vi "TestHarnessDPL-DetBoardOnly.vi"() -> ()   [LabVIEW 2025]
uses:
  <vilib>/Analysis/NI_AALBase.lvlib
  <userlib>/_OpenG.lib/time/time.llb/openg_time.lvlib
  <instrlib>/Detector SCPI/Detector SCPI.lvlib
  <vilib>/Analysis/1siggen.llb/Ramp Pattern by Delta.vi
  <instrlib>/Keithley 24XX/Keithley 24XX.lvlib
  <vilib>/Analysis/1siggen.llb/Ramp Pattern by Samples.vi
  <instrlib>/Keithley 648X Series/Keithley 648X Series.lvlib
  <vilib>/Analysis/NI_AALPro.lvlib
  <vilib>/Analysis/6fits.llb/Curve Fitting Criteria.ctl
  <vilib>/Utility/file.llb/Write Delimited Spreadsheet (DBL).vi
  <vilib>/Utility/file.llb/Write Delimited Spreadsheet (string).vi
panel:
  out "Array":dbl[][](array[numeric])
  out "BoardTemperature":dbl
  out "PicoAmmeter Resource":refnum<visa-resource-name>="Picoammeter"
  out "Searching":dbl[][](array[numeric])
  out "error out":errorcluster
  out "OpVsCurrent":cluster{"Ramp Pattern":dbl[], dbl[]}[](array[cluster])
  in  "Exit":bool
  in  "Measurement Mode":T1(tab)
  in  "test Results save directory":path
  in  "DetectorData":T2(array[cluster]) {"DAC Offset" min=1 max=4095 step=1}
  in  "SPI Clock":i64=10000000 format="%^.0e"
  in  "Oversample":i32=1 min=1 max=4096
  in  "Power":bool=TRUE
  in  "Detector VISA":refnum<visa-resource-name>="Detector_EGSE"
  out "Detector Resource":refnum<visa-resource-name>="COM4"
  out "Voltage (V)":dbl[](array[numeric])=[3.264, 0.0, 12.488, 12.77]
  out "Current (mA)":dbl[](array[numeric])=[0.0, 0.0, 21.6, -3.65]
  in  "ThrowAway":i32=100 min=1 max=10000
  out "Detector EGSE ID String":string="Aberystwyth University,Enfys Detector,#01,v0.5.0\r\n"
  in  "Current source":refnum<visa-resource-name>
  in  "Channel":u16(ring) items=["SWIR:High", "SWIR:Med", "SWIR:Low", "MWIR:High", "MWIR:Med", "MWIR:Low", "TRP:HSink", "TRP:SWIR"]
  in  "ReadMode":enum16{"Science", "Debug"}(ring)
  in  "Tab Control":T3(tab)
  out "Counts":dbl(graph)=160.194
  out "size":i32
  out "Elapsed(uS)":i32
  out "Mean Value (counts)":dbl
  out "rms (counts) 2":dbl=-2.7284841053187847e-12 format="%^.4g"
  out "Peak-to-Peak (counts)":dbl=0.0026870000001508743 format="%^.4g"
  in  "ResetVDACstats":bool
  out "Searching...":bool
  in  "Find Offset":bool
  in  "Target Counts":i32 min=0 max=4095
  in  "Tolerance":dbl
  in  "DAC Value":i32=2076 min=0 max=4095 step=1
  in  "Detector":u16(ring) items=["SWIR", "MWIR"]
  in  "Gain":u16(ring) items=["High", "Med", "Low"]
  in  "Export to Excel":bool
  in  "ResetScienceGraph":bool
  out "All Counts":T4(graph)
  out "Save FileName":string
  out "Temperature":dbl(graph)=160.194
  out "Waveform Chart":cluster{"output":i32, "output":i32}(graph)
  in  "Pause":bool
  out "XY Graph":cluster{dbl[], "subarray":dbl[]}(graph)
  in  "Detector 3":u16(ring) items=["SWIR", "MWIR"]
  in  "Gain 3":u16(ring) items=["High", "Med", "Low"]
  in  "trig":dbl=8.0 min=0.0 max=50.0
  in  "DetectorDAC":i32=2076 min=0 max=4095 step=1
  out "Output vs current":cluster{"Ramp Pattern":dbl[], dbl[]}[](graph)
  in  "ISweep":bool
  in  "NPoints":i32=10 min=10 max=10000 step=1
  in  "MaxCurrent":dbl=1e-11 min=1e-11 max=1e-06
  in  "MinCurrent":dbl=1e-12 min=-10.0 max=10.0
  in  "Detector 4":u16(ring) items=["SWIR", "MWIR"]
  in  "DecadeSweep":bool
  in  "Gain 4":u16(ring) items=["High", "Med", "Low"]
  out "slope (counts/nA)":dbl
  out "intercept":dbl
  out "residue":dbl
  out "Max Deviation (counts)":dbl
  in  "NumberDecades":i32
  in  "DAC":i32 min=0 max=4095 step=1
  in  "Modulation Steps":i32=2 min=2 max=1000 step=1
  in  "Modulation Max":dbl min=0.0 max=10.0
  in  "Modulation Min":dbl min=-10.0 max=10.0
  in  "SweepLight":bool
  in  "Detector 7":u16(ring) items=["SWIR", "MWIR"]
  out "Output vs Light":cluster{dbl[], dbl[]}[](graph)
  in  "Gain 2":u16(ring) items=["High", "Med", "Low"]
  in  "Abort 2":bool
  out "Output vs Light 2":cluster{dbl[], dbl[]}[](graph)
  in  "StopGathering":bool=TRUE
  in  "Detector 2":u16(ring) items=["SWIR", "MWIR"]
  out "PhotoDiode":dbl
  in  "millisecond multiple":u32
  in  "Manual LightSweep":bool
  in  "Tab Control 2":enum32{"Individual", "Science Mode"}(tab)
  out "VDAC Sweep":cluster{dbl[], dbl[]}[](graph)
  out "All Counts 2":cluster{"X-Data":dbl[], "SciData":dbl[]}[](graph)
  in  "SweepVDAC":bool
  in  "ISource":dbl min=-1e-06 max=1e-06
  in  "VDAC Step":i32=1 min=1 max=100
  in  "VDAC Max":i32 min=0 max=4095
  in  "VDAC Min":i32 min=0 max=4000
  in  "Channel":u16(ring) items=["SWIR", "MWIR"]
  in  "Abort SweepVDAC":bool
  in  "Step":bool
  in  "Delay 1 (ms)":i32
  in  "Current 2":dbl
  in  "Current 1":dbl
  out "Step Response":cluster{dbl[], "subarray":dbl[]}(graph)
  in  "chan (0)":i32
  out "exit":bool=TRUE
  # "3.3V supply"
  # "Heater"
  # "+12V Supply"
  # "-12V Supply"
  # "Pause button will halt collection and display.\nThis allows graph to be printed etc."
  # "Burst mode is intended to examine behaviour of the ADC\n\nA burst of readings is recorded on the EGSE and then gathered here."
  # "Light source modulated by USB205L working as voltage source connected to MOD input of LD250C\nreference photodiode monitored by 6846 picoammeter"
  # "Light source modulated by USB205L working as voltage source connected to MOD input of LD250C\nreference photodiode monitored by 6846 picoammeter"
  # "Set current to Current#1. Waits for Delay 1 to stabilise, then switches to current 2 and reads 1000 readings as fast as possible"
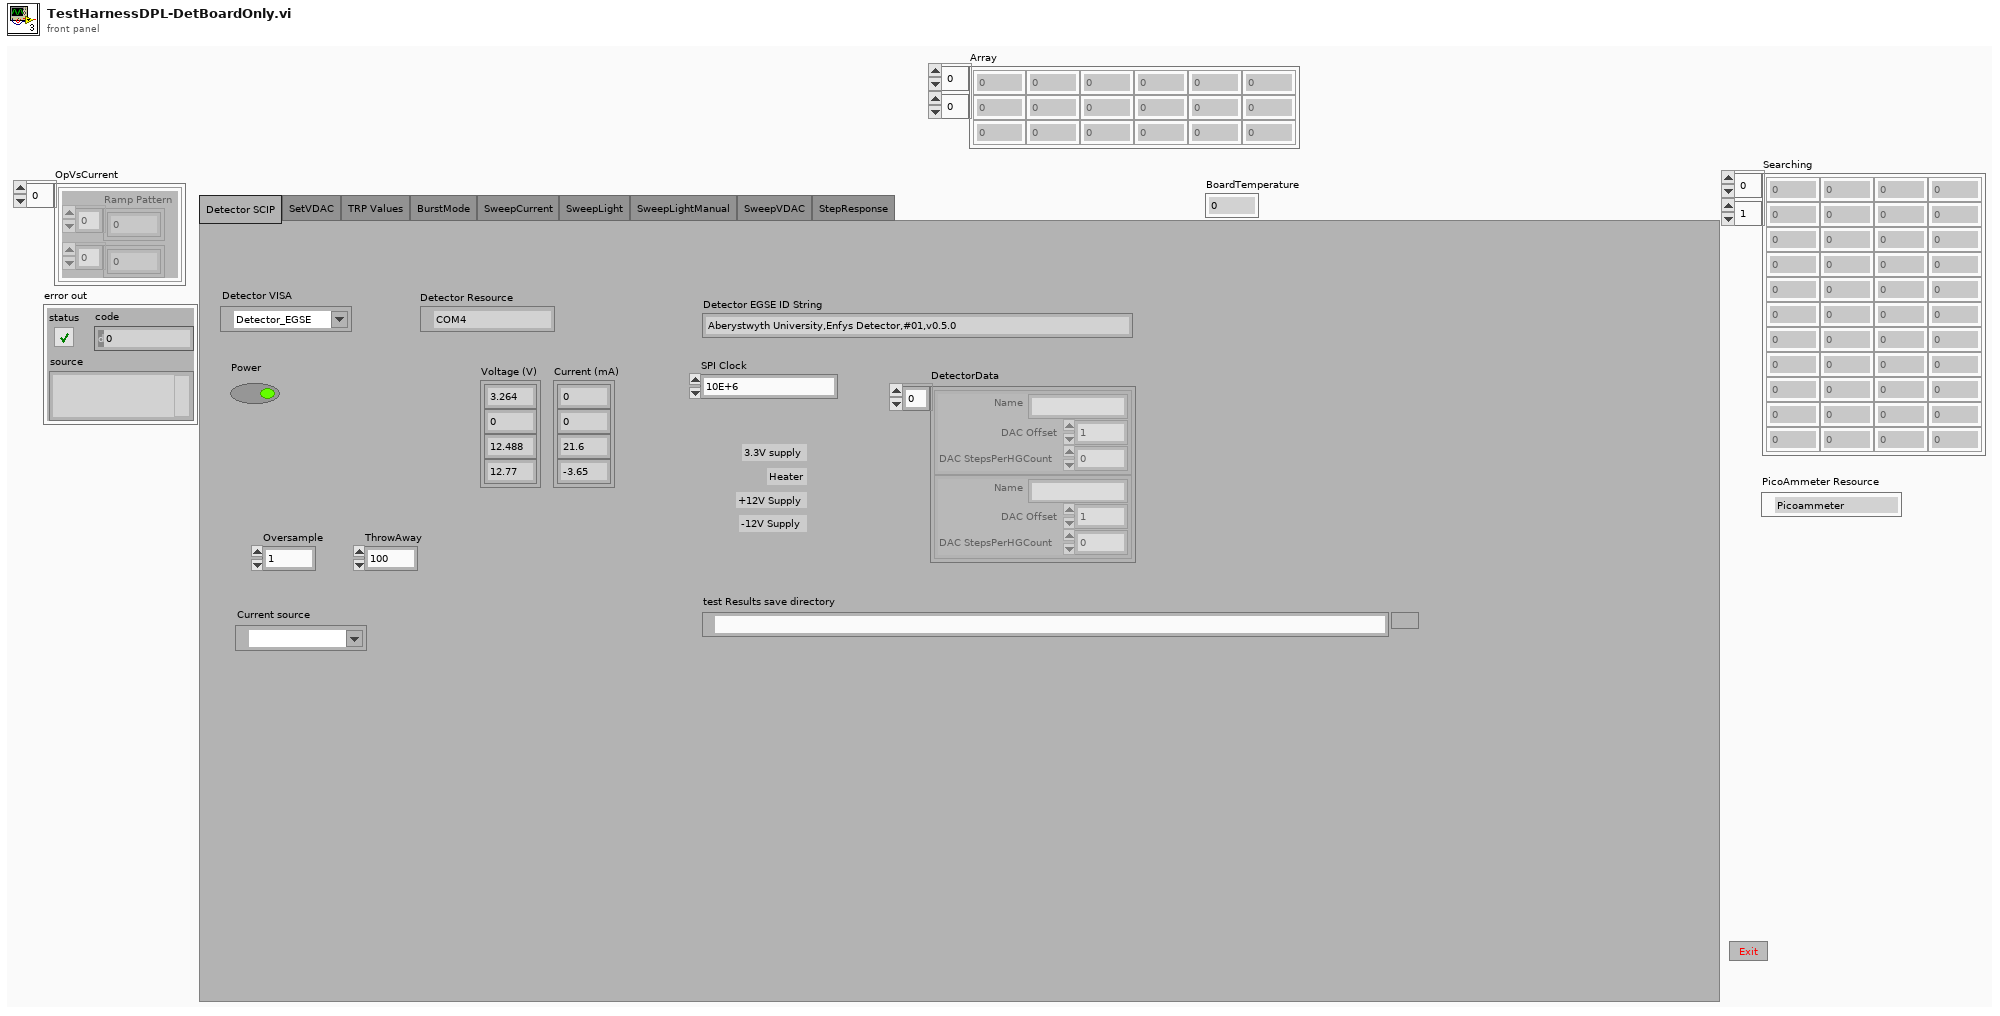
[diagram p1: front panel]
types:
  T1 = enum32{"Detector SCIP", "SetVDAC", "TRP Values", "BurstMode", "SweepCurrent", "SweepLight", "SweepLightManual", "SweepVDAC", "StepResponse"}
  T2 = cluster{"Name":string, "DAC Offset":i32, "DAC StepsPerHGCount":dbl}[]
  T3 = enum32{"Counts", "Science Packet", "Temperature"}
  T4 = cluster{"[0]":dbl, "[1]":dbl, "[2]":dbl, "[3]":dbl, "[4]":dbl, "[5]":dbl, "[6]":dbl, "[7]":dbl, "[8]":dbl, "[9]":dbl}
  T5 = cluster{"Baud Rate":u32, "Parity":u16, "Data Bits":u16, "Stop Bits":u16, "Flow Control":u16}
  T6 = cluster{"[0]":dbl, "[1]":dbl, "[2]":dbl, "[3]":dbl, "[4]":dbl, "[5]":dbl, "[6]":dbl, "[7]":dbl, "[8]":dbl, "[9]":dbl}[]
  T7 = cluster{"Name":string, "DAC Offset":i32, "DAC StepsPerHGCount":dbl}
  T8 = typedef "NI_AALPro.lvlib/Curve Fitting Criteria.ctl" = u16
  T9 = typedef "LVPointDoubleTypeDef.ctl" = cluster{"Cursor X":dbl, "Cursor Y":dbl}
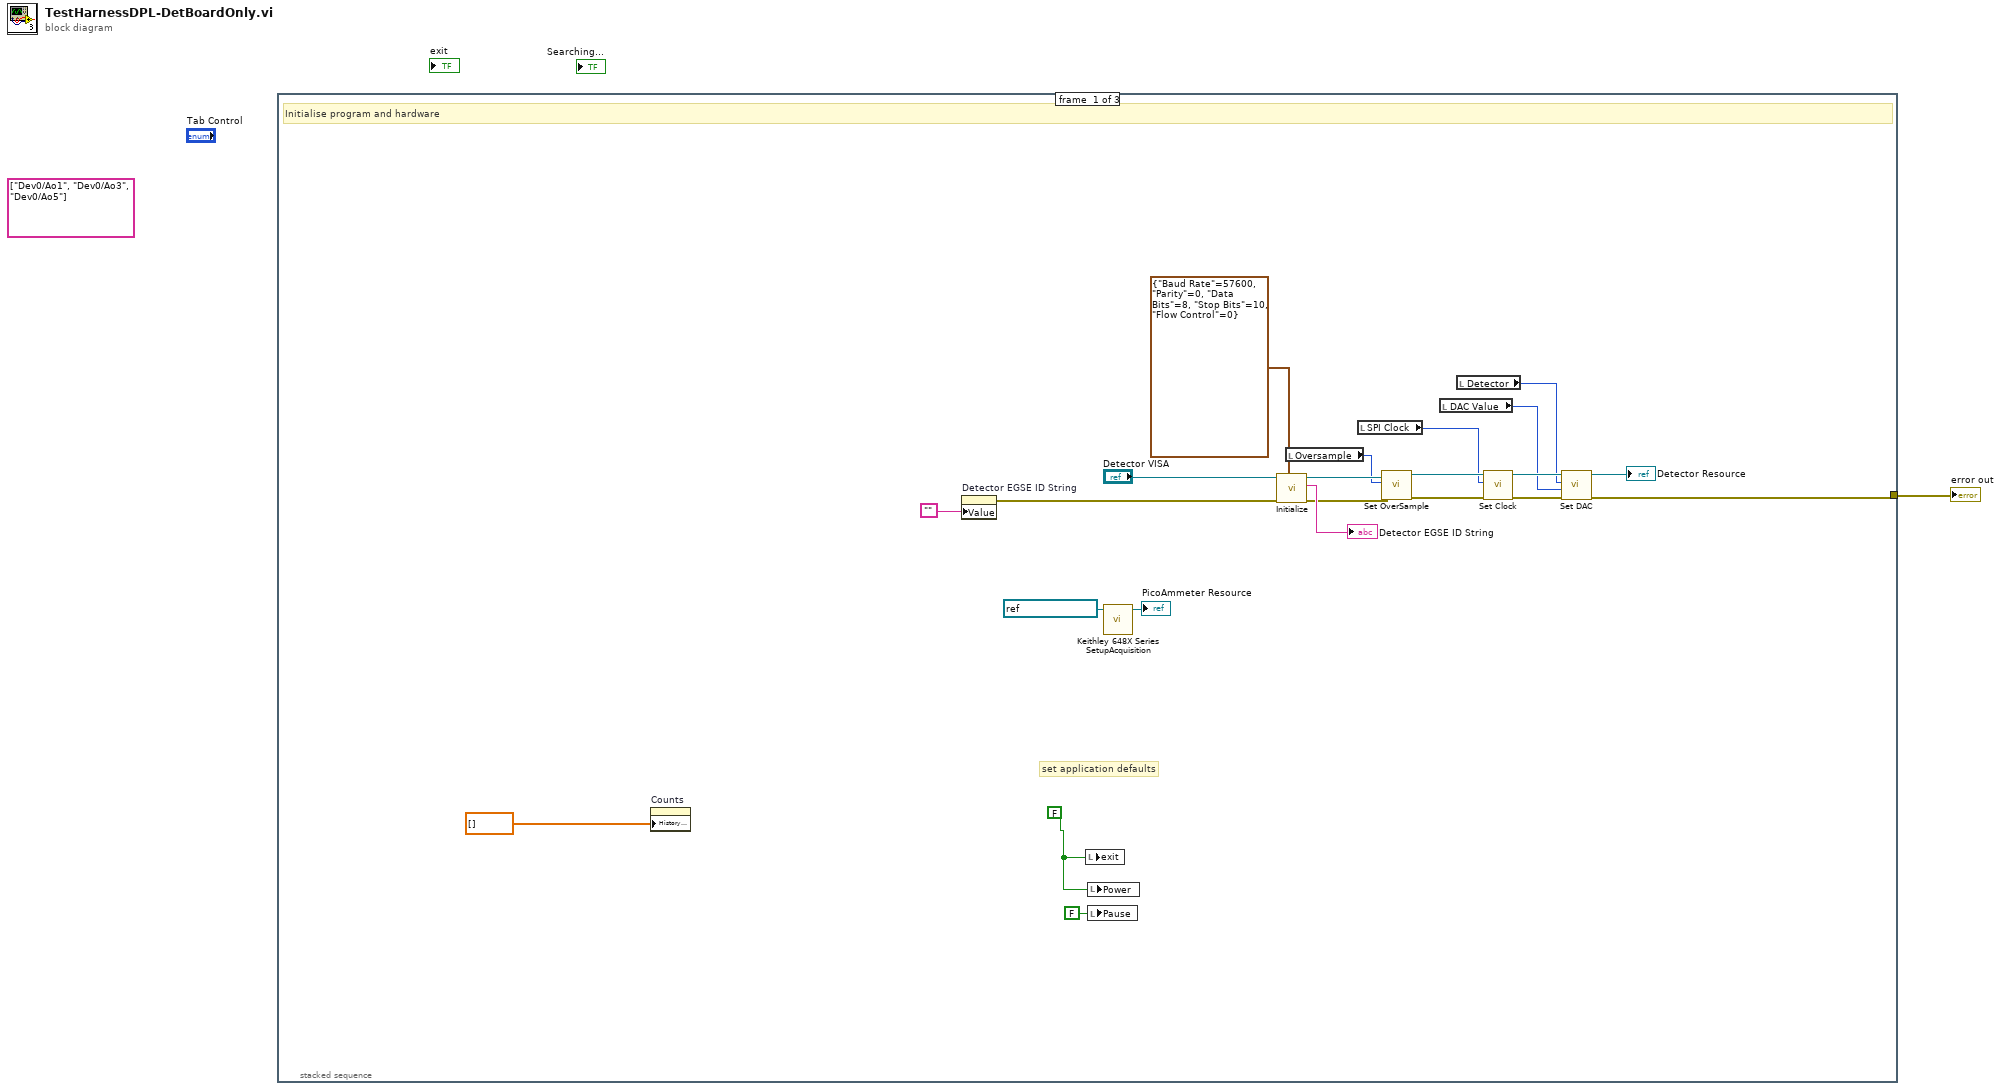
[diagram p0: block diagram]
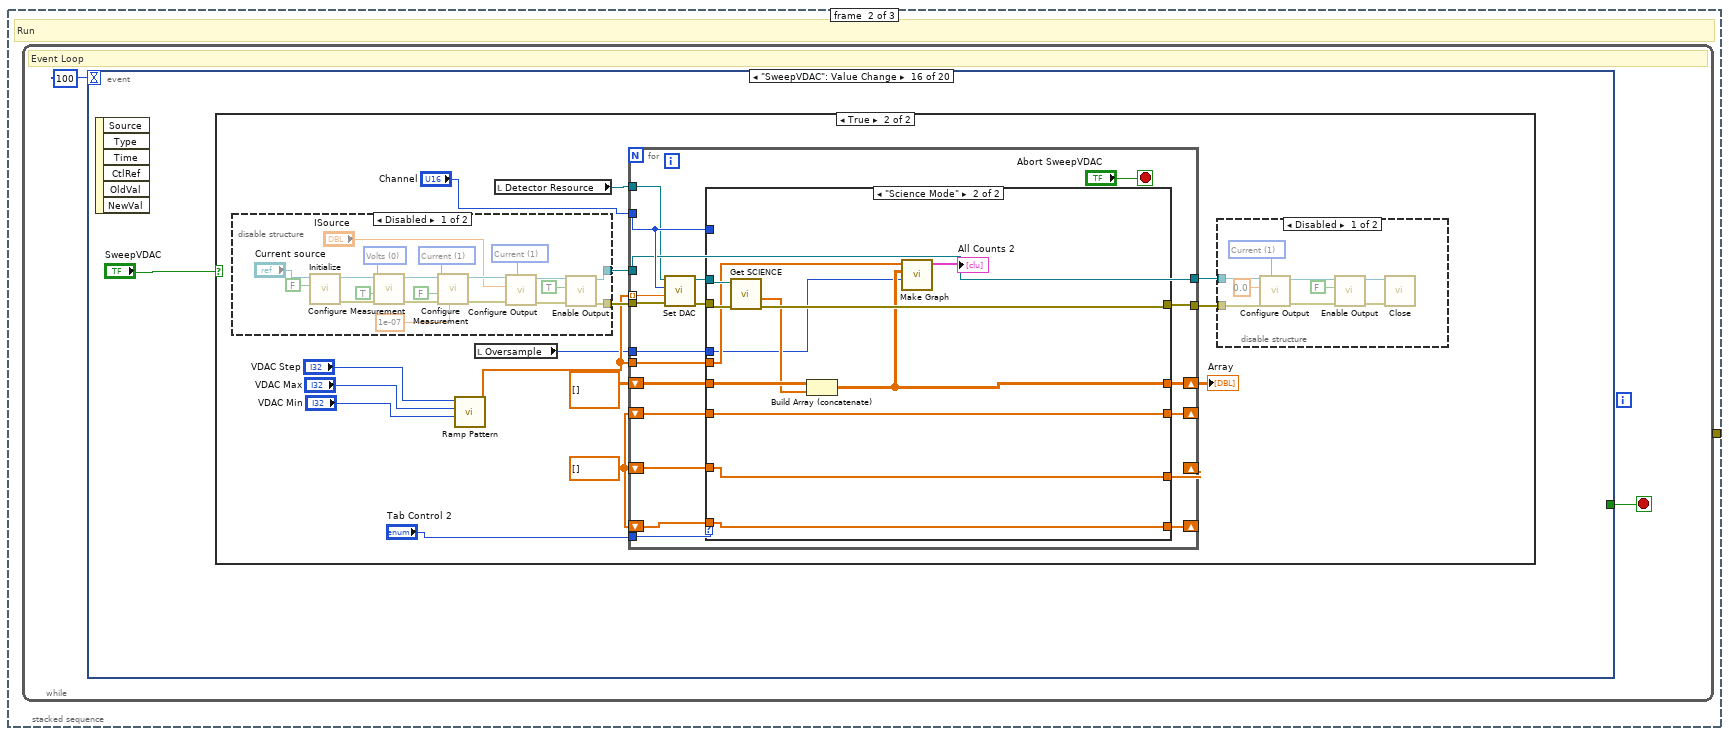
[diagram p2: hidden frame]
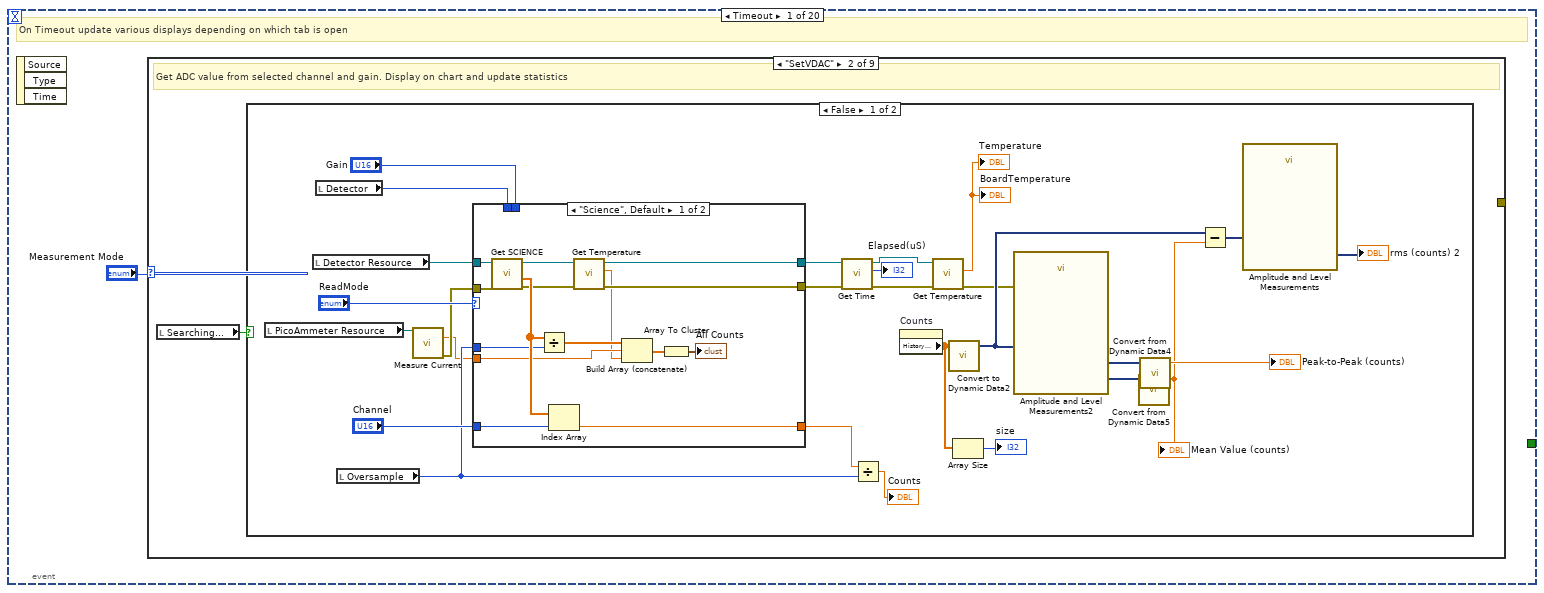
[diagram p3: hidden frame]
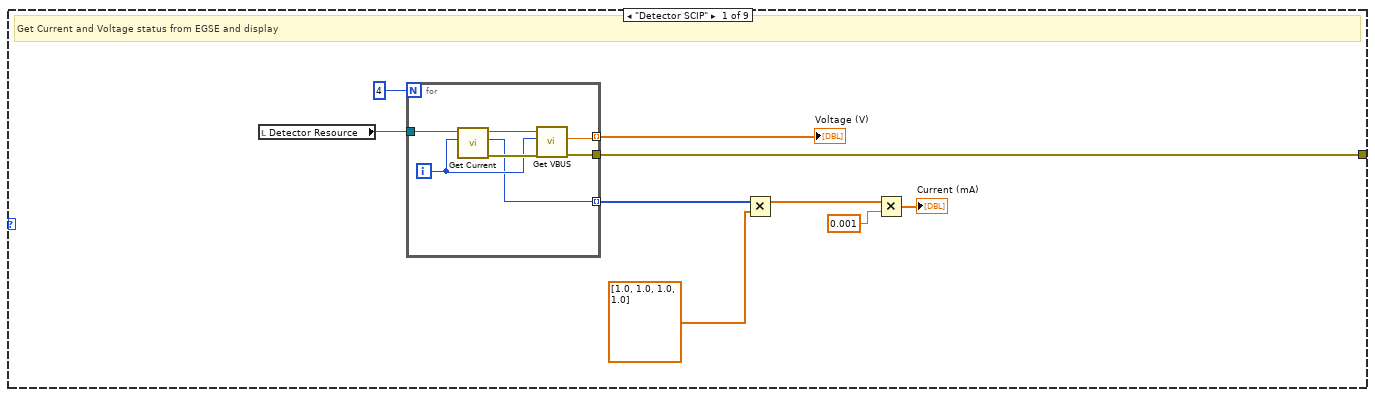
[diagram p4: hidden frame]
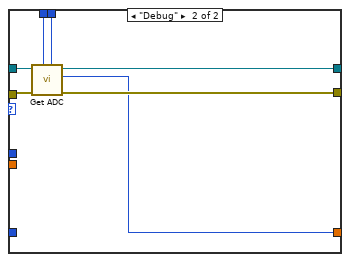
[diagram p5: hidden frame]
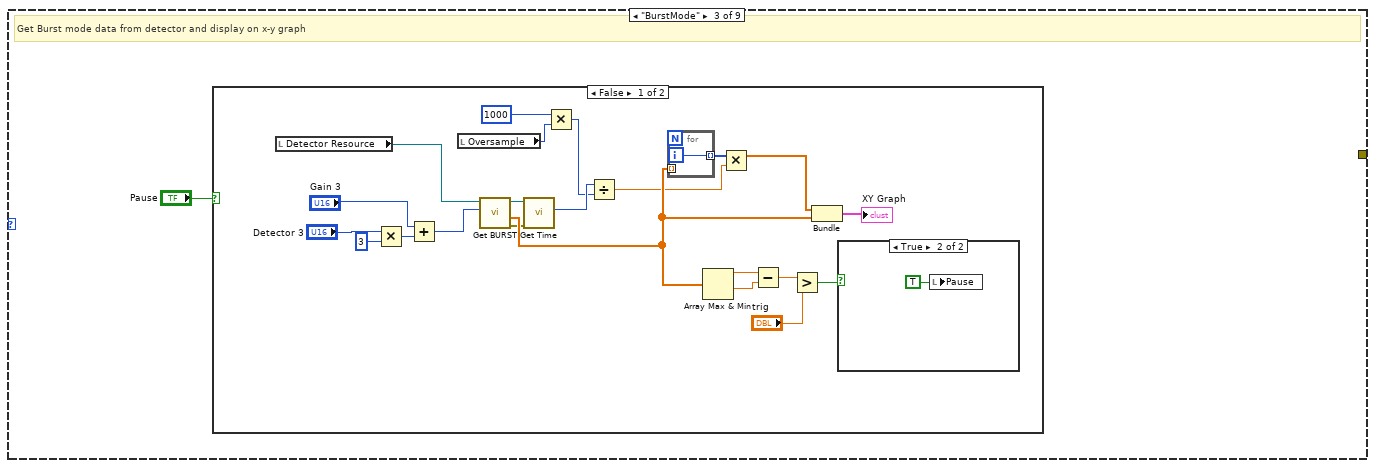
[diagram p7: hidden frame]
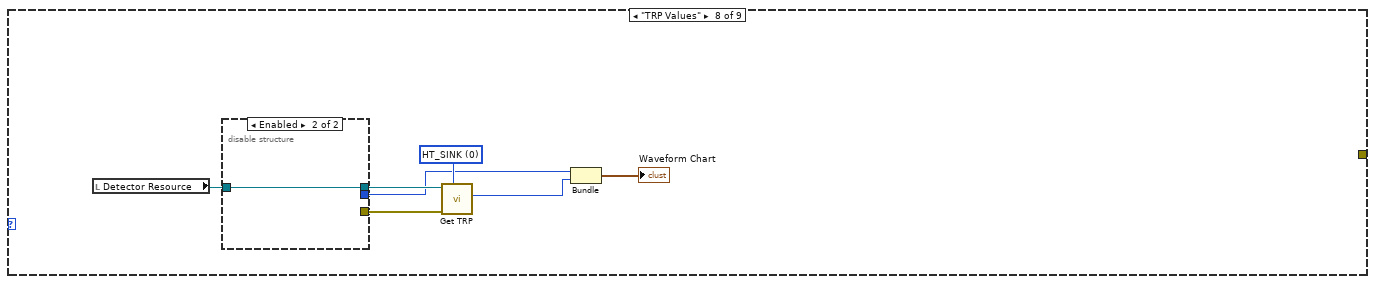
[diagram p14: hidden frame]
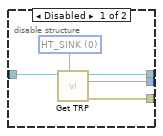
[diagram p15: hidden frame]
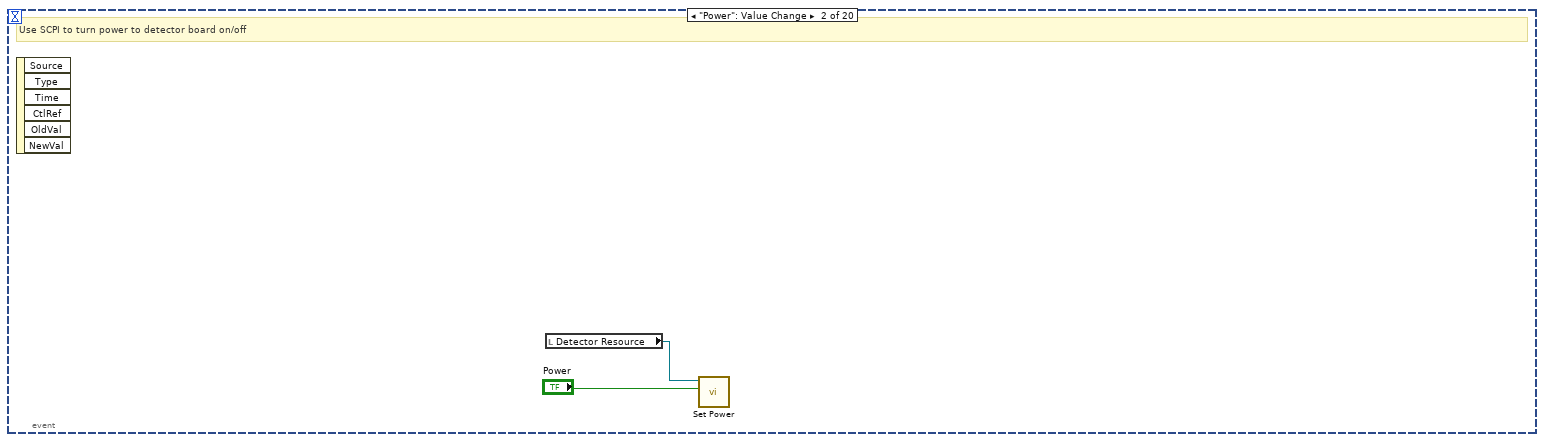
[diagram p17: hidden frame]
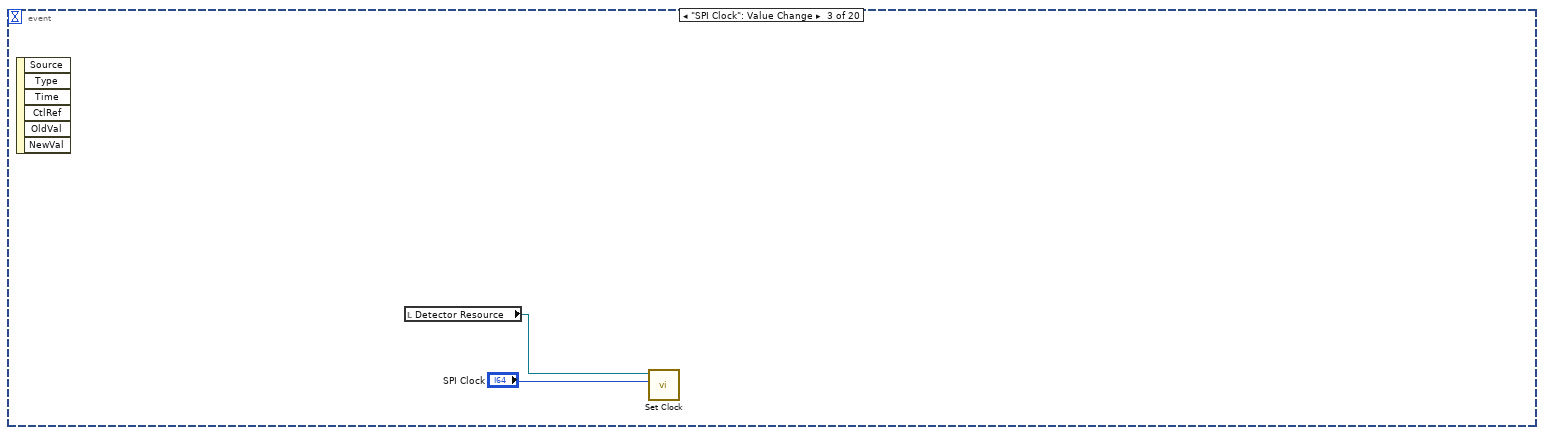
[diagram p18: hidden frame]
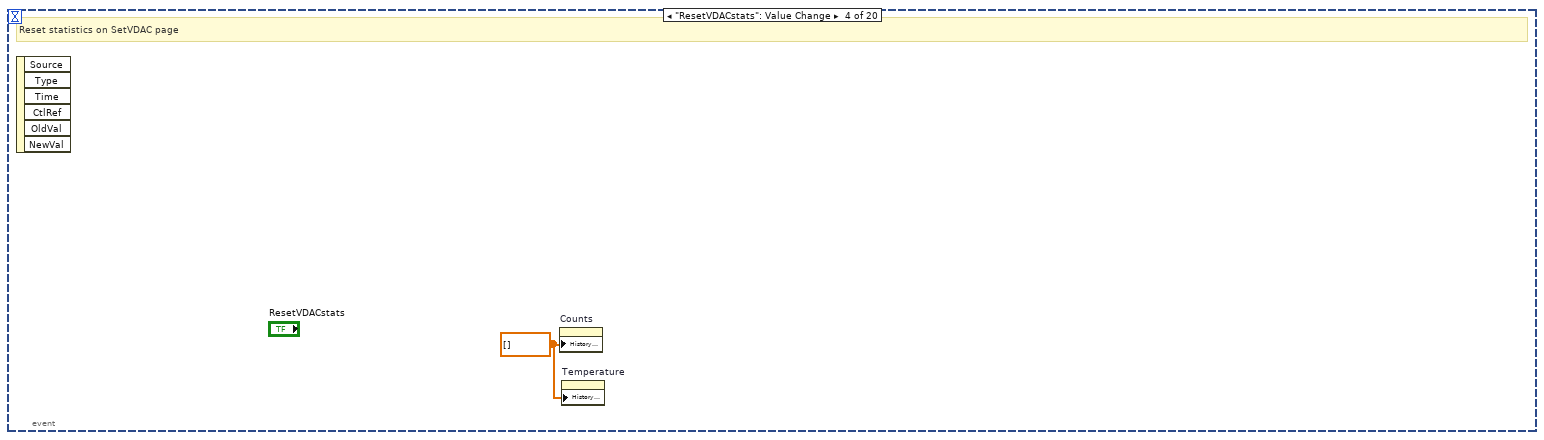
[diagram p19: hidden frame]
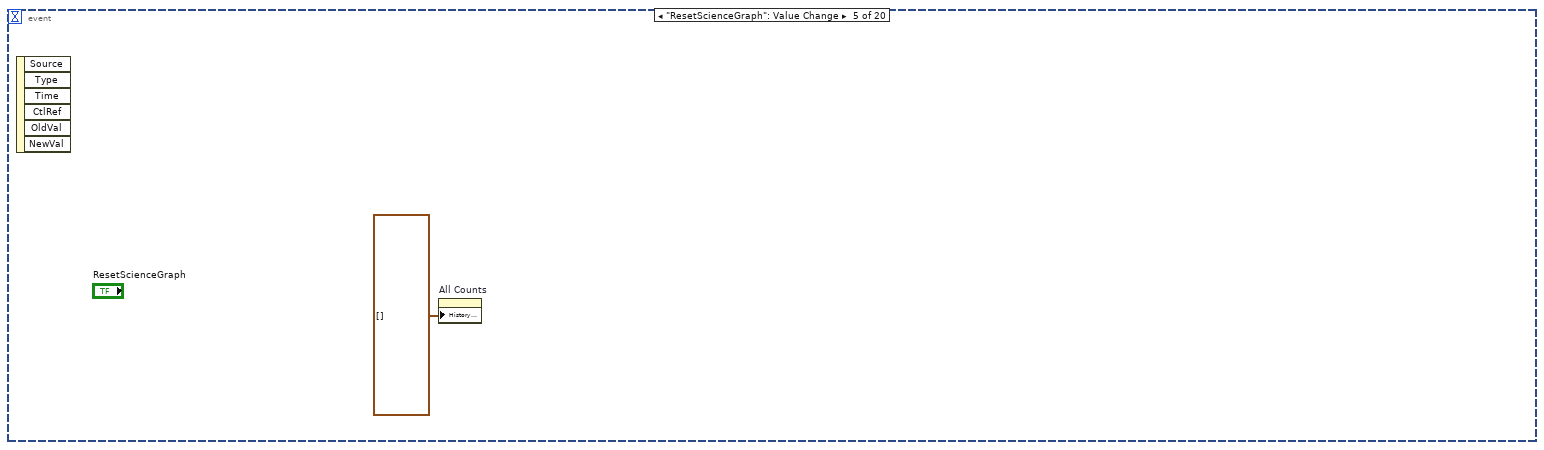
[diagram p20: hidden frame]
diagram:
  (unwired) string[] ["Dev0/Ao1", "Dev0/Ao3", "Dev0/Ao5"]
  n1 = stacked-sequence {
    tunnel: [w4 _ _] -> w1
    frame #0 {
      w22 = FALSE ("connected")
      # "set application defaults"
      # "Initialise program and hardware"
      n2 = property on="Counts" class="WFChart (strict)"("History Data"=dbl[] []) -> ()  [unwired: 2 in, 2 out]
      n3 = property on="Detector EGSE ID String" class="Str"("Value"="") -> (error out=w20:errorcluster)  [unwired: 2 in, 1 out]
      n4 = local write "exit"(w22) -> ()
      n5 = local write "Power"(w22) -> ()
      n6 = local write "Pause"(FALSE ("Pause")) -> ()
      n7 = call "Keithley 648X Series SetupAcquisition.vi"("VISA resource name"=refnum<visa-resource-name> "Picoammeter") -> ("VISA resource name out"=→"PicoAmmeter Resource":refnum<visa-resource-name>)  [unwired: 8 in, 1 out]
      n8 = call <instrlib>:"Initialize.vi"("Serial Configuration"=T5 {"Baud Rate"=57600, "Parity"=0, "Data Bits"=8, "Stop Bits"=10, "Flow Control"=0}, "error in (no error)"=w20, "VISA resource name"="Detector VISA") -> ("error out"=w16:errorcluster, "ID String"=→"Detector EGSE ID String":string, "VISA resource name out"=w15:refnum<visa-resource-name>)  [unwired: 6 in]
      n9 = local read "Oversample"() -> (w14:i32)
      n10 = local read "SPI Clock"() -> (w9:i64)
      n11 = call <instrlib>:"Set OverSample.vi"("error in (no error)"=w16, "oversample (0)"=w14, "VISA resource name"=w15) -> ("error out"=w13:errorcluster, "VISA resource name out"=w11:refnum<visa-resource-name>)  [unwired: 7 in]
      n12 = local read "DAC Value"() -> (w7:i32)
      n13 = local read "Detector"() -> (w8:u16)
      n14 = call <instrlib>:"Set Clock.vi"("error in (no error)"=w13, "ClockSpeed"=w9, "VISA resource name"=w11) -> ("error out"=w12:errorcluster, "VISA resource name out"=w10:refnum<visa-resource-name>)  [unwired: 7 in]
      n15 = call <instrlib>:"Set DAC.vi"("error in (no error)"=w12, "value (0)"=w7, "chan (0)"=w8, "VISA resource name"=w10) -> ("error out"=w4:errorcluster, "VISA resource name out"=→"Detector Resource":refnum<visa-resource-name>)  [unwired: 6 in]
    }
    frame #1 {
      # "Run"
      n16 = while {
        stop <- w24 stop-if-true
        # "Event Loop"
        n17 = event shown="[15] \"SweepVDAC\": Value Change" {
          selector: _ -> [_ _ _ _ _ _ _ _ _ _ _ _ _ _ _ _ _ _ _ _]
          dyn-events: _ -> [_ _ _ _ _ _ _ _ _ _ _ _ _ _ _ _ _ _ _ _]
          timeout: 100 -> [_ _ _ _ _ _ _ _ _ _ _ _ _ _ _ _ _ _ _ _]
          tunnel: [_ _ _ _ _ _ _ _ _ _ _ _ _ _ _ _ _ _ "Exit" _] -> w24
          event Timeout {
            # "On Timeout update various displays depending on which tab is open"
            n18 = event-data() -> ()  [unwired: 1 in, 3 out]
            n19 = case shown="\"SetVDAC\"" "Measurement Mode" {
              tunnel: [w27 _ _ _ _ _ _ _ _] -> _
              frame "Detector SCIP" {
                # "Get Current and Voltage status from EGSE and display"
                n20 = local read "Detector Resource"() -> (w35:refnum<visa-resource-name>)
                n21 = for {
                  N: 4 -> [_]
                  tunnel: w35 -> [w42]
                  tunnel: [w38] -> w32 mode=indexing
                  tunnel: [w37] -> w33 mode=indexing
                  tunnel: [w36] -> w27
                  i -> [w39]
                  n22 = call <instrlib>:"Get Current.vi"("chan (1)"=w39, "VISA resource name"=w42) -> ("error out"=w41:errorcluster, "output"=w38:i32, "VISA resource name out"=w40:refnum<visa-resource-name>)  [unwired: 7 in]
                  n23 = call <instrlib>:"Get VBUS.vi"("error in (no error)"=w41, "chan (1)"=w39, "VISA resource name"=w40) -> ("error out"=w36:errorcluster, "output"=w37:dbl)  [unwired: 6 in, 1 out]
                }
                "Voltage (V)" <- w33
                n24 = Multiply(x=w32, y=dbl[] [1.0, 1.0, 1.0, 1.0]) -> (x*y=w29:dbl[])
                n25 = Multiply(x=w29, y=0.001) -> (x*y=→"Current (mA)":dbl[])
              }
              frame "SetVDAC" {
                # "Get ADC value from selected channel and gain. Display on chart and update statistics"
                n26 = local read "Searching..."() -> (w43:bool)
                n27 = case shown="False" w43 {
                  frame False {
                    n28 = local read "PicoAmmeter Resource"() -> (w46:refnum<visa-resource-name>)
                    n29 = local read "Detector Resource"() -> (w70:refnum<visa-resource-name>)
                    n30 = local read "Detector"() -> (w68:u16)
                    n31 = local read "Oversample"() -> (w47:i32)
                    n32 = call <instrlib>:"Measure Current.vi"("VISA resource name"=w46) -> ("Measurement"=w44:dbl, "error out"=w45:errorcluster)  [unwired: 12 in, 1 out]
                    n33 = case shown="\"Science\", Default" "ReadMode" {
                      tunnel: w70 -> [w85 w92]
                      tunnel: "Gain" -> [_ w91]
                      tunnel: w68 -> [_ w90]
                      tunnel: [w72 w89] -> w67
                      tunnel: [w75 w88] -> w66
                      tunnel: [w83 w87] -> w48
                      tunnel: "Channel" -> [w84 _]
                      tunnel: w47 -> [w79 _]
                      tunnel: w45 -> [w78 w86]
                      tunnel: w44 -> [w76 _]
                      frame "Science", Default {
                        n34 = call <instrlib>:"Get SCIENCE.vi"("error in (no error)"=w78, "VISA resource name"=w85) -> ("error out"=w74:errorcluster, "subarray"=w80:dbl[], "VISA resource name out"=w73:refnum<visa-resource-name>)  [unwired: 6 in, 1 out]
                        n35 = Divide(x=w80, y=w79) -> (x/y=w81:dbl[])
                        n36 = Index Array(array=w80, index=w84) -> (element=w83:dbl)
                        n37 = call "Get Temperature.vi"("error in (no error)"=w74, "VISA resource name"=w73) -> ("error out"=w75:errorcluster, "output"=w71:dbl, "VISA resource name out"=w72:refnum<visa-resource-name>)  [unwired: 7 in]
                        n38 = Build Array (concatenate)(w81, w76, w71) -> (w77:dbl[])
                        n39 = Array To Cluster(array=w77) -> (cluster=→"All Counts":T4)
                      }
                      frame "Debug" {
                        n40 = call <instrlib>:"Get ADC.vi"("Gain"=w91, "Detector"=w90, "error in (no error)"=w86, "VISA resource name"=w92) -> ("error out"=w88:errorcluster, "output"=w87:i32, "VISA resource name out"=w89:refnum<visa-resource-name>)  [unwired: 5 in]
                      }
                    }
                    n41 = call <instrlib>:"Get Time.vi"("error in (no error)"=w66, "VISA resource name"=w67) -> ("error out"=w54:errorcluster, "output"=→"Elapsed(uS)":i32, "VISA resource name out"=w52:refnum<visa-resource-name>)  [unwired: 7 in]
                    n42 = Divide(x=w48, y=w47) -> (x/y=→"Counts":dbl)
                    n43 = property on="Counts" class="WFChart (strict)"() -> ("History Data"=w57:dbl[])  [unwired: 2 in, 2 out]
                    n44 = call "Get Temperature.vi"("error in (no error)"=w54, "VISA resource name"=w52) -> ("error out"=w53:errorcluster, "output"=→"Temperature" →"BoardTemperature":dbl)  [unwired: 7 in, 1 out]
                    n45 = call "Convert to Dynamic Data2"("Array"=w57) -> ("Dynamic Data Type"=w58:dynamicdata)  [unwired: 3 in]
                    n46 = Array Size(array=w57) -> (size(s)=→"size":i32)
                    n47 = call "Amplitude and Level Measurements2"("Signals"=w58, "error in (no error)"=w53) -> ("Mean (DC)"=w60:dynamicdata, "Peak to Peak"=w63:dynamicdata)  [unwired: 10 in, 2 out]
                    n48 = call "Convert from Dynamic Data5"("Dynamic Data Type"=w60) -> ("Scalar"=w59:dbl)  [unwired: 3 in]
                    "Mean Value (counts)" <- w59
                    n49 = call "Convert from Dynamic Data4"("Dynamic Data Type"=w63) -> ("Scalar"=→"Peak-to-Peak (counts)":dbl)  [unwired: 3 in]
                    n50 = Subtract(x=w58, y=w59) -> (x-y=w61:dynamicdata)
                    n51 = call "Amplitude and Level Measurements"("Signals"=w61) -> ("RMS"=→"rms (counts) 2":dynamicdata)  [unwired: 11 in, 3 out]
                  }
                  frame True {
                  }
                }
              }
              frame "BurstMode" {
                # "Get Burst mode data from detector and display on x-y graph"
                n52 = case shown="False" "Pause" {
                  frame False {
                    n53 = local read "Detector Resource"() -> (w115:refnum<visa-resource-name>)
                    n54 = Multiply(x="Detector 3", y=u16 3) -> (x*y=w114:u16)
                    n55 = Add(x="Gain 3", y=w114) -> (x+y=w112:u16)
                    n56 = local read "Oversample"() -> (w99:i32)
                    n57 = call <instrlib>:"Get BURST.vi"("chan (0)"=w112, "VISA resource name"=w115) -> ("error out"=w101:errorcluster, "subarray"=w107:dbl[], "VISA resource name out"=w100:refnum<visa-resource-name>)  [unwired: 6 in, 1 out]
                    n58 = call <instrlib>:"Get Time.vi"("error in (no error)"=w101, "VISA resource name"=w100) -> ("output"=w98:i32)  [unwired: 7 in, 2 out]
                    n59 = Multiply(x=1000, y=w99) -> (x*y=w95:i32)
                    n60 = Divide(x=w98, y=w95) -> (x/y=w96:dbl)
                    n61 = for {
                      tunnel: w107 -> [_] mode=indexing
                      tunnel: [w117] -> w108 mode=indexing
                      i -> [w117]
                    }
                    n62 = Array Max & Min(array=w107) -> (max value=w106:dbl, min value=w105:dbl)  [unwired: 2 out]
                    n63 = Multiply(x=w108, y=w96) -> (x*y=w97:dbl[])
                    n64 = Subtract(x=w106, y=w105) -> (x-y=w104:dbl)
                    n65 = Greater?(x=w104, y="trig") -> (0:w102:bool)
                    n66 = Bundle(w97, "subarray"=w107) -> (→"XY Graph":cluster{dbl[], "subarray":dbl[]})  [unwired: 1 in]
                    n67 = case shown="True" w102 {
                      frame False {
                      }
                      frame True {
                        n68 = local write "Pause"(TRUE ("Pause")) -> ()
                      }
                    }
                  }
                  frame True {
                  }
                }
              }
              frame "SweepCurrent" {
              }
              frame "SweepVDAC" {
              }
              frame "StepResponse" {
              }
              frame "SweepLight" {
              }
              frame "TRP Values" {
                w122 = u16 0 items=["HT_SINK", "SWIR_PCB"] ("TRP")
                n69 = local read "Detector Resource"() -> (w124:refnum<visa-resource-name>)
                n70 = disable-structure shown="Enabled" {
                  disable-tunnel: w124 -> [w129 w130]
                  disable-tunnel: [w127 w130] -> w123
                  disable-tunnel: [w126 _] -> w121
                  disable-tunnel: [w125 _] -> w120
                  frame Disabled {
                    w128 = u16 0 items=["HT_SINK", "SWIR_PCB"] ("TRP")
                    n71 = call <instrlib>:"Get TRP.vi"("TRP"=w128, "VISA resource name"=w129) -> ("error out"=w126:errorcluster, "output"=w125:i32, "VISA resource name out"=w127:refnum<visa-resource-name>)  [unwired: 7 in]
                  }
                  frame Enabled {
                  }
                }
                n72 = call <instrlib>:"Get TRP.vi"("TRP"=w122, "error in (no error)"=w121, "VISA resource name"=w123) -> ("output"=w119:i32)  [unwired: 6 in, 2 out]
                n73 = Bundle("output"=w120, "output"=w119) -> (→"Waveform Chart":cluster{"output":i32, "output":i32})  [unwired: 1 in]
              }
              frame "SweepLightManual" {
              }
            }
          }
          event "Power": Value Change {
            # "Use SCPI to turn power to detector board on/off"
            n74 = event-data() -> ()  [unwired: 1 in, 6 out]
            n75 = local read "Detector Resource"() -> (w132:refnum<visa-resource-name>)
            n76 = call <instrlib>:"Set Power.vi"("Power (0)"="Power", "VISA resource name"=w132) -> ()  [unwired: 8 in, 2 out]
          }
          event "SPI Clock": Value Change {
            n77 = event-data() -> ()  [unwired: 1 in, 6 out]
            n78 = local read "Detector Resource"() -> (w134:refnum<visa-resource-name>)
            n79 = call <instrlib>:"Set Clock.vi"("ClockSpeed"="SPI Clock", "VISA resource name"=w134) -> ()  [unwired: 8 in, 2 out]
          }
          event "ResetVDACstats": Value Change {
            w135 = dbl[] [] ("History Data")
            # "Reset statistics on SetVDAC page"
            n80 = event-data() -> ()  [unwired: 1 in, 6 out]
            n81 = property on="Counts" class="WFChart (strict)"("History Data"=w135) -> ()  [unwired: 2 in, 2 out]
            n82 = property on="Temperature" class="WFChart (strict)"("History Data"=w135) -> ()  [unwired: 2 in, 2 out]
          }
          event "ResetScienceGraph": Value Change {
            n83 = event-data() -> ()  [unwired: 1 in, 6 out]
            n84 = property on="All Counts" class="WFChart (strict)"("History Data"=T6 []) -> ()  [unwired: 2 in, 2 out]
          }
          event "Export to Excel": Value Change {
            w149 = "," ("delimiter (\\t)")
            n85 = event-data() -> ()  [unwired: 1 in, 6 out]
            n86 = Get Date/Time In Seconds() -> (seconds since 1Jan1904=w142:timestamp)
            n87 = Format Date/Time String(time format string (%c)="%Y%m%dT%H%M%S.csv", seconds (now)=w142) -> (date/time string=w139:string)  [unwired: 1 in]
            "Save FileName" <- w139
            n88 = Build Path(base path="test Results save directory", name or relative path=w139) -> (appended path=w138:path)
            n89 = for {
              N: 10 -> [_]
              tunnel: [w152] -> w145 mode=indexing
              i -> [w154]
              n90 = property on="All Counts" class="WFChart (strict)"("Active Plot"=w154) -> (error out=w153:errorcluster)  [unwired: 2 in, 1 out]
              n91 = property on="All Counts" class="WFChart (strict)"(error in=w153) -> ("Plot.Plot Name"=w152:string)  [unwired: 1 in, 2 out]
            }
            n92 = property on="All Counts" class="WFChart (strict)"() -> ("History Data"=w144:T6)  [unwired: 2 in, 2 out]
            n93 = for {
              tunnel: w144 -> [w151] mode=indexing
              tunnel: [w150] -> w147 mode=indexing
              n94 = Cluster To Array(cluster=w151) -> (array=w150:dbl[])
            }
            n95 = call-poly <vilib>:"Write Delimited Spreadsheet.vi"("file path (dialog if empty)"=w138, "1D data"=w145, "delimiter (\\t)"=w149) -> ("new file path (Not A Path if cancelled)"=w146:path)  [unwired: 11 in, 1 out]
            n96 = call-poly <vilib>:"Write Delimited Spreadsheet.vi"("file path (dialog if empty)"=w146, "format (%.3f)"="%.4g", "2D data"=w147, "append to file? (new file:F)"=TRUE, "delimiter (\\t)"=w149) -> ()  [unwired: 9 in, 2 out]
          }
          event "Oversample": Value Change {
            # "Change Oversample value on EGSE"
            n97 = event-data() -> ()  [unwired: 1 in, 6 out]
            n98 = local read "Detector Resource"() -> (w156:refnum<visa-resource-name>)
            n99 = call <instrlib>:"Set OverSample.vi"("oversample (0)"="Oversample", "VISA resource name"=w156) -> ()  [unwired: 8 in, 2 out]
          }
          event "ThrowAway": Value Change {
            # "Change Throwaway value on EGSE"
            n100 = event-data() -> ()  [unwired: 1 in, 6 out]
            n101 = local read "Detector Resource"() -> (w158:refnum<visa-resource-name>)
            n102 = call <instrlib>:"Set ThrowAway.vi"("ThrowAway (0)"="ThrowAway", "VISA resource name"=w158) -> ()  [unwired: 8 in, 2 out]
          }
          event "DAC Value": Value Change {
            # "Change offset DAC on selected channel of detector card and store new value in detecotr data"
            n103 = event-data() -> ()  [unwired: 1 in, 6 out]
            n104 = local read "Detector Resource"() -> (w165:refnum<visa-resource-name>)
            n105 = call <instrlib>:"Set DAC.vi"("value (0)"="DAC Value", "chan (0)"="Detector", "VISA resource name"=w165) -> ()  [unwired: 7 in, 2 out]
            n106 = local write "DetectorDAC"("DAC Value") -> ()
            n107 = Index Array(array="DetectorData", index="Detector") -> (element=w164:T7)
            n108 = Bundle By Name(cluster=w164, "DAC Offset"="DAC Value") -> (w161:T7)
            n109 = Replace Array Subset(array="DetectorData", new element=w161, index="Detector") -> (w160:T2)
            n110 = local write "DetectorData"(w160) -> ()
          }
          event "Detector": Value Change {
            n111 = event-data() -> ("NewVal"=w166:u16)  [unwired: 1 in, 5 out]
            n112 = local read "DetectorData"() -> (w169:T2)
            n113 = local write "Detector 4"(w166) -> ()
            n114 = Index Array(array=w169, index=w166) -> (element=w168:T7)
            n115 = Unbundle By Name(w168) -> ("DAC Offset"=w167:i32)
            n116 = local write "DAC Value"(w167) -> ()
            n117 = local write "DetectorDAC"(w167) -> ()
          }
          event "Detector 4": Value Change {
            n118 = event-data() -> ("NewVal"=w172:u16)  [unwired: 1 in, 5 out]
            n119 = local read "DetectorData"() -> (w173:T2)
            n120 = Index Array(array=w173, index=w172) -> (element=w171:T7)
            n121 = Unbundle By Name(w171) -> ("DAC Offset"=w170:i32)
            n122 = local write "DetectorDAC"(w170) -> ()
          }
          event "ISweep": Value Change {
            n123 = event-data() -> ()  [unwired: 1 in, 6 out]
            n124 = case shown="True" "ISweep" {
              frame False {
              }
              frame True {
                w183 = u16 50 items=["60 Hz"=60, "50 Hz or 400 Hz"=50] ("Power Line Frequency  (60 Hz)")
                w193 = u16 1 items=["Voltage", "Current"] ("Source Mode  (0: Voltage)")
                w202 = u16 1 items=["Volts", "Current", "Resistance"] ("Function (0: Volts)")
                w205 = u16 0 items=["Volts", "Current", "Resistance"] ("Function (0: Volts)")
                w209 = u16 1 items=["Voltage", "Current"] ("Source Mode  (0: Voltage)")
                w220 = dbl[] []
                n125 = call <instrlib>:"Initialize.vi"("ID Query (True)"=FALSE, "VISA resource name"=refnum<visa-resource-name> "B2901BL") -> ("error out"=w184:errorcluster, "VISA resource name out"=w187:refnum<visa-resource-name>)  [unwired: 8 in]
                n126 = call <instrlib>:"Configure Power Line Frequency.vi"("error in (no error)"=w184, "Power Line Frequency  (60 Hz)"=w183, "VISA resource name"=w187) -> ("error out"=w185:errorcluster, "VISA resource name out"=w186:refnum<visa-resource-name>)  [unwired: 7 in]
                n127 = call <instrlib>:"Configure Measurement.vi"("error in (no error)"=w185, "Enable Auto Range (T:Enable)"=TRUE, "Function (0: Volts)"=w205, "VISA resource name"=w186) -> ("error out"=w200:errorcluster, "VISA resource name out"=w201:refnum<visa-resource-name>)  [unwired: 6 in]
                n128 = call <instrlib>:"Configure Measurement.vi"("error in (no error)"=w200, "Enable Auto Range (T:Enable)"=TRUE, "Function (0: Volts)"=w202, "VISA resource name"=w201) -> ("error out"=w182:errorcluster, "VISA resource name out"=w181:refnum<visa-resource-name>)  [unwired: 6 in]
                n129 = local read "Detector Resource"() -> (w227:refnum<visa-resource-name>)
                n130 = VISA Write(VISA resource name=w181, write buffer=":SOUR:CURR:RANGE 1e-4", error in (no error)=w182) -> (VISA resource name out=w180:refnum<visa-resource-name>, error out=w179:errorcluster)  [unwired: 1 out]
                n131 = case shown="True" "DecadeSweep" {
                  tunnel: "MaxCurrent" -> [w231 _]
                  tunnel: "MinCurrent" -> [w230 w235]
                  tunnel: [w232 w234] -> w177
                  tunnel: "NumberDecades" -> [_ w236]
                  frame False {
                    n132 = call-poly <vilib>:"Ramp Pattern.vi"("start"=w230, "end"=w231, "samples"="NPoints") -> ("Ramp Pattern"=w232:dbl[])  [unwired: 7 in, 1 out]
                  }
                  frame True {
                    n133 = call "Decades125.vi"("BaseUnit"=w235, "NumberDecades"=w236) -> ("output array"=w234:dbl[])  [unwired: 9 in]
                  }
                }
                n134 = call <instrlib>:"Configure Output.vi"("Source Mode  (0: Voltage)"=w209, "error in (no error)"=w179, "Output Level (0)"=0.0, "VISA resource name"=w180) -> ("error out"=w208:errorcluster, "VISA resource name out"=w207:refnum<visa-resource-name>)  [unwired: 6 in]
                n135 = local read "Gain 4"() -> (w212:u16)
                n136 = call <instrlib>:"Enable Output.vi"("error in (no error)"=w208, "Enable Output (T: Enable)"=TRUE ("Auto Output-Off (F: Disable)"), "VISA resource name"=w207) -> ("error out"=w198:errorcluster, "VISA resource name out"=w197:refnum<visa-resource-name>)  [unwired: 7 in]
                n137 = call <instrlib>:"Set DAC.vi"("error in (no error)"=w198, "value (0)"="DetectorDAC", "chan (0)"="Detector 4", "VISA resource name"=w227) -> ("error out"=w222:errorcluster, "VISA resource name out"=w226:refnum<visa-resource-name>)  [unwired: 6 in]
                n138 = local read "Oversample"() -> (w228:i32)
                n139 = property on="Gain" class="Ring (strict)"() -> (error out=w213:errorcluster, "Strings []"=w218:string[])  [unwired: 2 in, 1 out]
                n140 = call <userlib>:"Wait (ms)__ogtk.vi"("error in (no error)"=w222, "milliseconds to wait"=u32 1000) -> ("error out"=w223:errorcluster)  [unwired: 8 in, 1 out]
                n141 = Index Array(array=w218, index=w212) -> (element=w214:string)
                n142 = for {
                  tunnel: w223 -> [w250]
                  tunnel: w177 -> [w239] mode=indexing
                  tunnel: [w248] -> w188
                  shift-right: [w255] -> _
                  shift-left: w220 -> [w257]
                  tunnel: w177 -> [w243]
                  tunnel: w226 -> [w254]
                  tunnel: w228 -> [w252]
                  tunnel: "Detector 4" -> [w251]
                  tunnel: [w249] -> w189
                  tunnel: [w241] -> w219
                  tunnel: w220 -> [w242]
                  tunnel: w197 -> [w237]
                  w238 = u16 1 items=["Voltage", "Current"] ("Source Mode  (0: Voltage)")
                  n143 = call <instrlib>:"Configure Output.vi"("Source Mode  (0: Voltage)"=w238, "error in (no error)"=w250, "Output Level (0)"=w239, "VISA resource name"=w237) -> ("error out"=w247:errorcluster, "VISA resource name out"=w249:refnum<visa-resource-name>)  [unwired: 6 in]
                  n144 = call <userlib>:"Wait Until Next ms Multiple__ogtk.vi"("error in (no error)"=w247, "milliseconds to wait"=u32 100) -> ("error out"=w246:errorcluster)  [unwired: 8 in, 1 out]
                  n145 = call <instrlib>:"Get ADC.vi"("Gain"="Gain 4", "Detector"=w251, "error in (no error)"=w246, "VISA resource name"=w254) -> ("error out"=w248:errorcluster, "output"=w256:i32)  [unwired: 5 in, 1 out]
                  n146 = Divide(x=w256, y=w252) -> (x/y=w253:dbl)
                  n147 = Build Array (concatenate)(w257, w253) -> (w255:dbl[])
                  n148 = Bundle("output array"=w243, w255) -> (w244:cluster{"output array":dbl[], dbl[]})  [unwired: 1 in]
                  n149 = Bundle("output array"=w243, w242) -> (w240:cluster{"output array":dbl[], dbl[]})  [unwired: 1 in]
                  n150 = Build Array(w244, w240) -> (w241:cluster{"output array":dbl[], dbl[]}[])
                  "Output vs current" <- w241
                }
                "OpVsCurrent" <- w219
                n151 = property on="Output vs current" class="XYGraph (strict)"(error in=w213, "Active Plot"=u32 0) -> (error out=w215:errorcluster)  [unwired: 1 in, 1 out]
                n152 = property on="Output vs current" class="XYGraph (strict)"(error in=w215, "Plot.Plot Name"=w214) -> ()  [unwired: 1 in, 2 out]
                n153 = call <instrlib>:"Configure Output.vi"("Source Mode  (0: Voltage)"=w193, "error in (no error)"=w188, "Output Level (0)"=0.0, "VISA resource name"=w189) -> ("error out"=w191:errorcluster, "VISA resource name out"=w190:refnum<visa-resource-name>)  [unwired: 6 in]
                n154 = call <instrlib>:"Enable Output.vi"("error in (no error)"=w191, "Enable Output (T: Enable)"=FALSE ("Auto Output-Off (F: Disable)"), "VISA resource name"=w190) -> ("error out"=w195:errorcluster, "VISA resource name out"=w196:refnum<visa-resource-name>)  [unwired: 7 in]
                n155 = call <instrlib>:"Close.vi"("error in (no error)"=w195, "VISA resource name"=w196) -> ()  [unwired: 9 in, 1 out]
              }
            }
          }
          event "Output vs current": Cursor Release {
            w277 = T8 0 items=["Least Square", "Least Absolute Residual", "Bisquare"] ("method")
            n156 = event-data() -> ()  [unwired: 1 in, 9 out]
            n157 = property on="Output vs current" class="XYGraph (strict)"("Active Cursor"=u32 0) -> (error out=w289:errorcluster)  [unwired: 2 in, 1 out]
            n158 = property on="Output vs current" class="XYGraph (strict)"(error in=w289) -> (error out=w286:errorcluster, "Cursor.Cursor Position"=w284:T9)  [unwired: 1 in, 1 out]
            n159 = Unbundle By Name(w284) -> ("Cursor X"=w272:dbl)
            n160 = local read "OpVsCurrent"() -> (w285:cluster{"Ramp Pattern":dbl[], dbl[]}[])
            n161 = property on="Output vs current" class="XYGraph (strict)"(error in=w286, "Active Cursor"=u32 1) -> (error out=w288:errorcluster)  [unwired: 1 in, 1 out]
            n162 = Index Array(array=w285) -> (element=w269:cluster{"Ramp Pattern":dbl[], dbl[]})  [unwired: 1 in]
            n163 = property on="Output vs current" class="XYGraph (strict)"(error in=w288) -> ("Cursor.Cursor Position"=w283:T9)  [unwired: 1 in, 2 out]
            n164 = Unbundle(w269) -> ("Ramp Pattern"=w282:dbl[], w280:dbl[])
            n165 = Unbundle By Name(w283) -> ("Cursor X"=w273:dbl)
            n166 = Max & Min(x=w273, y=w272) -> (max(x,y)=w270:dbl, min(x,y)=w271:dbl)
            n167 = Search 1D Array(1D array=w282, element=w271) -> (index of element=w279:i32)  [unwired: 1 in]
            n168 = local read "Output vs current"() -> (w267:cluster{"Ramp Pattern":dbl[], dbl[]}[])
            n169 = Search 1D Array(1D array=w282, element=w270) -> (index of element=w281:i32)  [unwired: 1 in]
            n170 = Subtract(x=w281, y=w279) -> (x-y=w278:i32)
            n171 = Array Subset(array=w280, index=w279, length=w278) -> (w262:dbl[])
            n172 = Array Subset(array=w282, index=w279, length=w278) -> (w268:dbl[])
            n173 = call <vilib>:"Linear Fit.vi"("Y"=w262, "X"=w268, "method"=w277) -> ("Best Linear Fit"=w263:dbl[], "slope"=→"slope (counts/nA)":dbl, "intercept"=→"intercept":dbl, "residue"=→"residue":dbl)  [unwired: 8 in, 1 out]
            n174 = Bundle(w268, "Best Linear Fit"=w263) -> (w265:cluster{dbl[], "Best Linear Fit":dbl[]})  [unwired: 1 in]
            n175 = Replace Array Subset(array=w267, new element=w265, index=1) -> (w264:cluster{"Ramp Pattern":dbl[], dbl[]}[])
            n176 = Subtract(x=w262, y=w263) -> (x-y=w261:dbl[])
            n177 = local write "Output vs current"(w264) -> ()
            n178 = Absolute Value(x=w261) -> (abs(x)=w260:dbl[])
            n179 = Array Max & Min(array=w260) -> (max value=→"Max Deviation (counts)":dbl)  [unwired: 3 out]
          }
          event "SweepLight": Value Change {
            n180 = event-data() -> ()  [unwired: 1 in, 6 out]
            n181 = case shown="True" "SweepLight" {
              frame False {
              }
              frame True {
                w308 = dbl[] []
                n182 = disable-structure shown="Disabled" {
                  disable-tunnel: [w318 _] -> w309
                  frame Disabled {
                    n183 = call "Keithley 648X Series SetupAcquisition.vi"("VISA resource name"=refnum<visa-resource-name> "Picoammeter") -> ("VISA resource name out"=w318:refnum<visa-resource-name>)  [unwired: 8 in, 1 out]
                  }
                  frame Enabled {
                  }
                }
                n184 = local read "Detector Resource"() -> (w316:refnum<visa-resource-name>)
                n185 = local read "Oversample"() -> (w317:i32)
                n186 = call-poly <vilib>:"Ramp Pattern.vi"("start"="Modulation Min", "end"="Modulation Max", "samples"="Modulation Steps") -> ("Ramp Pattern"=w312:dbl[])  [unwired: 7 in, 1 out]
                n187 = call <instrlib>:"Set DAC.vi"("value (0)"="DAC", "chan (0)"="Detector 7", "VISA resource name"=w316) -> ("error out"=w307:errorcluster, "VISA resource name out"=w315:refnum<visa-resource-name>)  [unwired: 7 in]
                n188 = call <instrlib>:"ULx Create Channel (AO-Voltage-Basic).vi"("maximum value"=5.0, "minimum value"=0.0, "physical channels"=refnum<k21> "Dev0/Ao0", "error in"=w307) -> ("task out"=w302:refnum<k24>, "error out"=w301:errorcluster)  [unwired: 10 in]
                n189 = call <instrlib>:"ULx Write (Analog 1D DBL 1Chan 1Samp).vi"("task in"=w302, "data"="Modulation Min", "error in"=w301) -> ("task out"=w303:refnum<k24>, "error out"=w298:errorcluster)  [unwired: 10 in, 1 out]
                n190 = call <userlib>:"Wait (ms)__ogtk.vi"("error in (no error)"=w298, "milliseconds to wait"=u32 1000) -> ("error out"=w299:errorcluster)  [unwired: 8 in, 1 out]
                n191 = for {
                  tunnel: w299 -> [w348]
                  tunnel: [w347] -> w293
                  tunnel: [w329] -> w295
                  shift-right: [w342] -> _
                  shift-left: w308 -> [w344]
                  tunnel: w315 -> [w341]
                  shift-right: [w337] -> _
                  shift-left: w308 -> [w339]
                  shift-right: [w336] -> _
                  shift-left: w308 -> [w338]
                  tunnel: w317 -> [w331]
                  tunnel: "Detector 7" -> [w330]
                  tunnel: w312 -> [w322] mode=indexing
                  tunnel: w309 -> [w328]
                  shift-right: [w324] -> _
                  shift-left: w308 -> [w325]
                  tunnel: w303 -> [w323]
                  stop <- "Abort 2" stop-if-true
                  n192 = call <instrlib>:"ULx Write (Analog 1D DBL 1Chan 1Samp).vi"("task in"=w323, "data"=w322, "error in"=w348) -> ("task out"=w347:refnum<k24>, "error out"=w346:errorcluster)  [unwired: 10 in, 1 out]
                  n193 = call <instrlib>:"Get ADC.vi"("Gain"="Gain 2", "Detector"=w330, "error in (no error)"=w346, "VISA resource name"=w341) -> ("error out"=w340:errorcluster, "output"=w343:i32)  [unwired: 5 in, 1 out]
                  n194 = Divide(x=w343, y=w331) -> (x/y=w320:dbl)
                  n195 = Divide(x=w330, y=w331) -> ()  [unwired: 1 out]
                  n196 = Build Array (concatenate)(w339, w320) -> (w337:dbl[])
                  n197 = Build Array (concatenate)(w344, w320) -> (w342:dbl[])
                  n198 = Build Array (concatenate)(w338, w320) -> (w336:dbl[])
                  n199 = call <instrlib>:"Measure Current.vi"("VISA resource name"=w328, "error in (no error)"=w340) -> ("Measurement"=w326:dbl, "error out"=w329:errorcluster)  [unwired: 11 in, 1 out]
                  n200 = Negate(x=w326) -> (-x=w321:dbl)
                  n201 = Build Array (concatenate)(w325, w321) -> (w324:dbl[])
                  n202 = Bundle(w324, w342) -> (w335:cluster{dbl[], dbl[]})  [unwired: 1 in]
                  n203 = Bundle(w324, w337) -> (w334:cluster{dbl[], dbl[]})  [unwired: 1 in]
                  n204 = Bundle(w324, w336) -> (w333:cluster{dbl[], dbl[]})  [unwired: 1 in]
                  n205 = Build Array(w335, w334, w333) -> (→"Output vs Light":cluster{dbl[], dbl[]}[])
                }
                n206 = call <instrlib>:"ULx Write (Analog 1D DBL 1Chan 1Samp).vi"("task in"=w293, "data"=0.0, "error in"=w295) -> ("task out"=w294:refnum<k24>, "error out"=w296:errorcluster)  [unwired: 10 in, 1 out]
                n207 = call <instrlib>:"ULx Clear Task.vi"("task in"=w294, "error in"=w296) -> ()  [unwired: 13 in, 1 out]
              }
            }
          }
          event "Manual LightSweep": Value Change {
            n208 = event-data() -> ()  [unwired: 1 in, 6 out]
            n209 = case shown="True" "Manual LightSweep" {
              frame False {
              }
              frame True {
                w355 = dbl[] []
                n210 = property on="Measurement Mode" class="TabCtl (strict)"("Value"=T1."SweepLightManual" ("Measurement Mode")) -> (error out=w354:errorcluster)  [unwired: 2 in, 1 out]
                n211 = local read "PicoAmmeter Resource"() -> (w350:refnum<visa-resource-name>)
                n212 = local read "Detector Resource"() -> (w357:refnum<visa-resource-name>)
                n213 = local read "Oversample"() -> (w356:i32)
                n214 = while {
                  tunnel: [w388] -> w351
                  shift-right: [w391] -> _
                  shift-left: w355 -> [w393]
                  shift-right: [w381] -> _
                  shift-left: w355 -> [w383]
                  shift-right: [w380] -> _
                  shift-left: w355 -> [w382]
                  tunnel: "Detector 2" -> [w371]
                  tunnel: w357 -> [w370]
                  tunnel: w356 -> [w369]
                  tunnel: w350 -> [w366]
                  shift-right: [w363] -> _
                  shift-left: w355 -> [w365]
                  tunnel: [w361] -> _
                  tunnel: w354 -> [w360]
                  stop <- "StopGathering" stop-if-true
                  w384 = u16 2 items=["High", "Med", "Low"] ("Gain")
                  w385 = u16 1 items=["High", "Med", "Low"] ("Gain")
                  w394 = u16 0 items=["High", "Med", "Low"] ("Gain")
                  n215 = flat-sequence {
                    tunnel: w360 -> [w395]
                    tunnel: [w395] -> w359
                    frame #0 {
                      n216 = Wait Until Next ms Multiple(millisecond multiple="millisecond multiple") -> ()  [unwired: 1 out]
                    }
                  }
                  n217 = call <instrlib>:"Measure Current.vi"("VISA resource name"=w366, "error in (no error)"=w359) -> ("VISA resource name out"=w361:refnum<visa-resource-name>, "Measurement"=w364:dbl, "error out"=w367:errorcluster)  [unwired: 11 in]
                  "PhotoDiode" <- w364
                  n218 = Build Array (concatenate)(w365, w364) -> (w363:dbl[])
                  n219 = call <instrlib>:"Get ADC.vi"("Gain"=w394, "Detector"=w371, "error in (no error)"=w367, "VISA resource name"=w370) -> ("error out"=w390:errorcluster, "output"=w392:i32, "VISA resource name out"=w387:refnum<visa-resource-name>)  [unwired: 5 in]
                  n220 = Divide(x=w392, y=w369) -> (x/y=w372:dbl)
                  n221 = call <instrlib>:"Get ADC.vi"("Gain"=w385, "Detector"=w371, "error in (no error)"=w390, "VISA resource name"=w387) -> ("error out"=w389:errorcluster, "output"=w376:i32, "VISA resource name out"=w386:refnum<visa-resource-name>)  [unwired: 5 in]
                  n222 = Divide(x=w376, y=w369) -> (x/y=w373:dbl)
                  n223 = call <instrlib>:"Get ADC.vi"("Gain"=w384, "Detector"=w371, "error in (no error)"=w389, "VISA resource name"=w386) -> ("error out"=w388:errorcluster, "output"=w375:i32)  [unwired: 5 in, 1 out]
                  n224 = Divide(x=w375, y=w369) -> (x/y=w374:dbl)
                  n225 = Build Array (concatenate)(w383, w373) -> (w381:dbl[])
                  n226 = Build Array (concatenate)(w393, w372) -> (w391:dbl[])
                  n227 = Build Array (concatenate)(w382, w374) -> (w380:dbl[])
                  n228 = Bundle(w363, w391) -> (w379:cluster{dbl[], dbl[]})  [unwired: 1 in]
                  n229 = Bundle(w363, w381) -> (w378:cluster{dbl[], dbl[]})  [unwired: 1 in]
                  n230 = Bundle(w363, w380) -> (w377:cluster{dbl[], dbl[]})  [unwired: 1 in]
                  n231 = Build Array(w379, w378, w377) -> (→"Output vs Light 2":cluster{dbl[], dbl[]}[])
                }
                n232 = property on="StopGathering" class="Bool (strict)"(error in=w351, "Value"=FALSE ("StopGathering")) -> ()  [unwired: 1 in, 2 out]
              }
            }
          }
          event "SweepVDAC": Value Change {
            n233 = event-data() -> ()  [unwired: 1 in, 6 out]
            n234 = case shown="True" "SweepVDAC" {
              frame False {
              }
              frame True {
                w408 = dbl[] []
                n235 = disable-structure shown="Disabled" {
                  disable-tunnel: [w428 _] -> w412
                  disable-tunnel: [w427 _] -> w411
                  frame Disabled {
                    w432 = u16 1 items=["Voltage", "Current"] ("Source Mode  (0: Voltage)")
                    w436 = u16 1 items=["Volts", "Current", "Resistance"] ("Function (0: Volts)")
                    w438 = u16 0 items=["Volts", "Current", "Resistance"] ("Function (0: Volts)")
                    n236 = call <instrlib>:"Initialize.vi"("ID Query (True)"=FALSE, "VISA resource name"="Current source") -> ("error out"=w425:errorcluster, "VISA resource name out"=w426:refnum<visa-resource-name>)  [unwired: 8 in]
                    n237 = call <instrlib>:"Configure Measurement.vi"("error in (no error)"=w425, "Enable Auto Range (T:Enable)"=TRUE, "Function (0: Volts)"=w438, "VISA resource name"=w426) -> ("error out"=w439:errorcluster, "VISA resource name out"=w440:refnum<visa-resource-name>)  [unwired: 6 in]
                    n238 = call <instrlib>:"Configure Measurement.vi"("Manual Range (1.0)"=1e-07, "error in (no error)"=w439, "Enable Auto Range (T:Enable)"=FALSE, "Function (0: Volts)"=w436, "VISA resource name"=w440) -> ("error out"=w434:errorcluster, "VISA resource name out"=w433:refnum<visa-resource-name>)  [unwired: 5 in]
                    n239 = call <instrlib>:"Configure Output.vi"("Source Mode  (0: Voltage)"=w432, "error in (no error)"=w434, "Output Level (0)"="ISource", "VISA resource name"=w433) -> ("error out"=w431:errorcluster, "VISA resource name out"=w430:refnum<visa-resource-name>)  [unwired: 6 in]
                    n240 = call <instrlib>:"Enable Output.vi"("error in (no error)"=w431, "Enable Output (T: Enable)"=TRUE, "VISA resource name"=w430) -> ("error out"=w427:errorcluster, "VISA resource name out"=w428:refnum<visa-resource-name>)  [unwired: 7 in]
                  }
                  frame Enabled {
                  }
                }
                n241 = call-poly <vilib>:"Ramp Pattern.vi"("start"="VDAC Min", "end"="VDAC Max", "delta"="VDAC Step") -> ("Ramp Pattern"=w410:dbl[])  [unwired: 6 in, 2 out]
                n242 = local read "Oversample"() -> (w407:i32)
                n243 = local read "Detector Resource"() -> (w409:refnum<visa-resource-name>)
                n244 = for {
                  tunnel: w412 -> [w447]
                  tunnel: w411 -> [w461]
                  tunnel: w410 -> [w460] mode=indexing
                  tunnel: [w447] -> w406
                  tunnel: [w456] -> w405
                  shift-right: [w457] -> _
                  shift-left: w408 -> [w458]
                  tunnel: w410 -> [w451]
                  tunnel: w409 -> [w446]
                  shift-right: [w453] -> _
                  shift-left: w408 -> [w455]
                  shift-right: [w452] -> _
                  shift-left: w408 -> [w454]
                  tunnel: w407 -> [w449]
                  tunnel: "Channel" -> [w448]
                  tunnel: "Tab Control 2" -> [w444]
                  shift-right: [w442] -> w399
                  shift-left: dbl[][] [] -> [w443]
                  stop <- "Abort SweepVDAC" stop-if-true
                  n245 = call <instrlib>:"Set DAC.vi"("error in (no error)"=w461, "value (0)"=w460, "chan (0)"=w448, "VISA resource name"=w446) -> ("error out"=w459:errorcluster, "VISA resource name out"=w445:refnum<visa-resource-name>)  [unwired: 6 in]
                  n246 = case shown="\"Science Mode\"" w444 {
                    tunnel: w459 -> [w491 w502]
                    tunnel: w458 -> [w489 w500]
                    tunnel: [w487 w500] -> w457
                    tunnel: [w484 w501] -> w456
                    tunnel: w455 -> [w479 w499]
                    tunnel: w454 -> [w478 w498]
                    tunnel: [w477 w499] -> w453
                    tunnel: [w476 w498] -> w452
                    tunnel: w451 -> [w475 w495]
                    tunnel: w449 -> [w469 w492]
                    tunnel: w448 -> [w467 _]
                    tunnel: w445 -> [w466 w503]
                    tunnel: w443 -> [w462 w497]
                    tunnel: [w462 w493] -> w442
                    frame "Individual", Default {
                      w480 = u16 2 items=["High", "Med", "Low"] ("Gain")
                      w481 = u16 1 items=["High", "Med", "Low"] ("Gain")
                      w490 = u16 0 items=["High", "Med", "Low"] ("Gain")
                      n247 = call <instrlib>:"Get ADC.vi"("Gain"=w490, "Detector"=w467, "error in (no error)"=w491, "VISA resource name"=w466) -> ("error out"=w486:errorcluster, "output"=w488:i32, "VISA resource name out"=w483:refnum<visa-resource-name>)  [unwired: 5 in]
                      n248 = Divide(x=w488, y=w469) -> (x/y=w463:dbl)
                      n249 = call <instrlib>:"Get ADC.vi"("Gain"=w481, "Detector"=w467, "error in (no error)"=w486, "VISA resource name"=w483) -> ("error out"=w485:errorcluster, "output"=w470:i32, "VISA resource name out"=w482:refnum<visa-resource-name>)  [unwired: 5 in]
                      n250 = Divide(x=w470, y=w469) -> (x/y=w464:dbl)
                      n251 = call <instrlib>:"Get ADC.vi"("Gain"=w480, "Detector"=w467, "error in (no error)"=w485, "VISA resource name"=w482) -> ("error out"=w484:errorcluster, "output"=w468:i32)  [unwired: 5 in, 1 out]
                      n252 = Divide(x=w468, y=w469) -> (x/y=w465:dbl)
                      n253 = Build Array (concatenate)(w479, w464) -> (w477:dbl[])
                      n254 = Build Array (concatenate)(w489, w463) -> (w487:dbl[])
                      n255 = Build Array (concatenate)(w478, w465) -> (w476:dbl[])
                      n256 = Bundle("Ramp Pattern"=w475, w487) -> (w474:cluster{"Ramp Pattern":dbl[], dbl[]})  [unwired: 1 in]
                      n257 = Bundle("Ramp Pattern"=w475, w477) -> (w473:cluster{"Ramp Pattern":dbl[], dbl[]})  [unwired: 1 in]
                      n258 = Bundle("Ramp Pattern"=w475, w476) -> (w472:cluster{"Ramp Pattern":dbl[], dbl[]})  [unwired: 1 in]
                      n259 = Build Array(w474, w473, w472) -> (→"VDAC Sweep":cluster{"Ramp Pattern":dbl[], dbl[]}[])
                    }
                    frame "Science Mode" {
                      n260 = call <instrlib>:"Get SCIENCE.vi"("error in (no error)"=w502, "VISA resource name"=w503) -> ("error out"=w501:errorcluster, "subarray"=w494:dbl[])  [unwired: 6 in, 2 out]
                      n261 = Build Array (concatenate)(w497, w494) -> (w493:dbl[][])
                      n262 = call "Make Graph.vi"(9:w492, "SciData"=w493, "X-Data"=w495) -> ("All Counts 2"=→"All Counts 2":cluster{"X-Data":dbl[], "SciData":dbl[]}[])  [unwired: 8 in]
                    }
                  }
                }
                "Array" <- w399
                n263 = disable-structure shown="Disabled" {
                  disable-tunnel: w406 -> [w417 _]
                  disable-tunnel: w405 -> [w415 _]
                  frame Disabled {
                    w418 = u16 1 items=["Voltage", "Current"] ("Source Mode  (0: Voltage)")
                    n264 = call <instrlib>:"Configure Output.vi"("Source Mode  (0: Voltage)"=w418, "error in (no error)"=w415, "Output Level (0)"=0.0, "VISA resource name"=w417) -> ("error out"=w414:errorcluster, "VISA resource name out"=w416:refnum<visa-resource-name>)  [unwired: 6 in]
                    n265 = call <instrlib>:"Enable Output.vi"("error in (no error)"=w414, "Enable Output (T: Enable)"=FALSE, "VISA resource name"=w416) -> ("error out"=w420:errorcluster, "VISA resource name out"=w419:refnum<visa-resource-name>)  [unwired: 7 in]
                    n266 = call <instrlib>:"Close.vi"("error in (no error)"=w420, "VISA resource name"=w419) -> ()  [unwired: 9 in, 1 out]
                  }
                  frame Enabled {
                  }
                }
              }
            }
          }
          event "Step": Value Change {
            n267 = event-data() -> ()  [unwired: 1 in, 6 out]
            n268 = case shown="True" "Step" {
              frame False {
              }
              frame True {
                w516 = 1000 ("oversample (0)")
                w528 = u16 1 items=["Voltage", "Current"] ("Source Mode  (0: Voltage)")
                w532 = u16 1 items=["Voltage", "Current"] ("Source Mode  (0: Voltage)")
                w535 = u16 1 items=["Volts", "Current", "Resistance"] ("Function (0: Volts)")
                w538 = u16 0 items=["Volts", "Current", "Resistance"] ("Function (0: Volts)")
                n269 = local read "Detector Resource"() -> (w512:refnum<visa-resource-name>)
                n270 = property on="Oversample" class="DigNum (strict)"() -> (error out=w524:errorcluster, "Value"=w507:i32)  [unwired: 2 in, 1 out]
                n271 = call <instrlib>:"Set OverSample.vi"("error in (no error)"=w524, "oversample (0)"=w516, "VISA resource name"=w512) -> ("error out"=w525:errorcluster)  [unwired: 7 in, 1 out]
                n272 = local read "Current source"() -> (w505:refnum<visa-resource-name>)
                n273 = call <instrlib>:"Initialize.vi"("error in (no error)"=w525, "ID Query (True)"=FALSE, "VISA resource name"=w505) -> ("error out"=w548:errorcluster, "VISA resource name out"=w547:refnum<visa-resource-name>)  [unwired: 7 in]
                n274 = call <instrlib>:"Configure Measurement.vi"("error in (no error)"=w548, "Enable Auto Range (T:Enable)"=TRUE, "Function (0: Volts)"=w538, "VISA resource name"=w547) -> ("error out"=w542:errorcluster, "VISA resource name out"=w541:refnum<visa-resource-name>)  [unwired: 6 in]
                n275 = call <instrlib>:"Configure Measurement.vi"("Manual Range (1.0)"=1e-07, "error in (no error)"=w542, "Enable Auto Range (T:Enable)"=FALSE, "Function (0: Volts)"=w535, "VISA resource name"=w541) -> ("error out"=w543:errorcluster, "VISA resource name out"=w544:refnum<visa-resource-name>)  [unwired: 5 in]
                n276 = call <instrlib>:"Configure Output.vi"("Source Mode  (0: Voltage)"=w532, "error in (no error)"=w543, "Output Level (0)"="Current 1", "VISA resource name"=w544) -> ("error out"=w545:errorcluster, "VISA resource name out"=w546:refnum<visa-resource-name>)  [unwired: 6 in]
                n277 = call <instrlib>:"Enable Output.vi"("error in (no error)"=w545, "Enable Output (T: Enable)"=TRUE, "VISA resource name"=w546) -> ("error out"=w531:errorcluster, "VISA resource name out"=w527:refnum<visa-resource-name>)  [unwired: 7 in]
                n278 = call <userlib>:"Wait (ms)__ogtk.vi"("error in (no error)"=w531, "milliseconds to wait"="Delay 1 (ms)") -> ("error out"=w529:errorcluster)  [unwired: 8 in, 1 out]
                n279 = call <instrlib>:"Configure Output.vi"("Source Mode  (0: Voltage)"=w528, "error in (no error)"=w529, "Output Level (0)"="Current 2", "VISA resource name"=w527) -> ("error out"=w523:errorcluster, "VISA resource name out"=w509:refnum<visa-resource-name>)  [unwired: 6 in]
                n280 = call <instrlib>:"Get BURST.vi"("error in (no error)"=w523, "chan (0)"="chan (0)", "VISA resource name"=w512) -> ("error out"=w521:errorcluster, "subarray"=w514:dbl[], "VISA resource name out"=w520:refnum<visa-resource-name>)  [unwired: 5 in, 1 out]
                n281 = for {
                  tunnel: w514 -> [_] mode=indexing
                  tunnel: [w549] -> w519 mode=indexing
                  i -> [w549]
                }
                n282 = call <instrlib>:"Get Time.vi"("error in (no error)"=w521, "VISA resource name"=w520) -> ("error out"=w510:errorcluster, "output"=w518:i32, "VISA resource name out"=w506:refnum<visa-resource-name>)  [unwired: 7 in]
                n283 = Divide(x=w518, y=w516) -> (x/y=w517:dbl)
                n284 = Multiply(x=w517, y=w519) -> (x*y=w515:dbl[])
                n285 = Bundle(w515, "subarray"=w514) -> (→"Step Response":cluster{dbl[], "subarray":dbl[]})  [unwired: 1 in]
                n286 = call <instrlib>:"Enable Output.vi"("error in (no error)"=w510, "Enable Output (T: Enable)"=TRUE, "VISA resource name"=w509) -> ("error out"=w508:errorcluster)  [unwired: 7 in, 1 out]
                n287 = call <instrlib>:"Set OverSample.vi"("error in (no error)"=w508, "oversample (0)"=w507, "VISA resource name"=w506) -> ()  [unwired: 7 in, 2 out]
              }
            }
          }
          event "Find Offset": Value Change {
            n288 = event-data() -> ()  [unwired: 1 in, 6 out]
            n289 = local read "Detector Resource"() -> (w556:refnum<visa-resource-name>)
            n290 = property on="Searching..." class="Bool (strict)"("Value"=TRUE ("Searching...")) -> (error out=w562:errorcluster)  [unwired: 2 in, 1 out]
            n291 = local read "Detector"() -> (w557:u16)
            n292 = while {
              shift-right: [w574] -> _
              shift-left: 4095 -> [w569]
              shift-right: [w573] -> _
              shift-left: 1 -> [w570]
              tunnel: w562 -> [w579]
              tunnel: [w565] -> w559
              tunnel: w557 -> [w576]
              tunnel: w556 -> [w575]
              tunnel: [w572] -> w554 mode=indexing
              tunnel: [w571] -> w555 mode=indexing
              tunnel: [w564] -> w553 mode=indexing
              tunnel: [w567] -> w550 mode=indexing
              stop <- w580 stop-if-true
              n293 = Subtract(x=w569, y=w570) -> (x-y=w582:i32)
              n294 = Absolute Value(x=w582) -> (abs(x)=w578:i32)
              n295 = Less Or Equal?(x=w578, y=1) -> (x <= y?=w581:bool)
              n296 = case shown="False" w581 {
                tunnel: w569 -> [w595 w631]
                tunnel: w570 -> [w594 w633]
                tunnel: [w593 w633] -> w573
                tunnel: [w596 TRUE] -> w580
                tunnel: w579 -> [w607 _]
                tunnel: [w591 w631] -> w574
                tunnel: [w590 _] -> w566
                tunnel: w576 -> [w588 _]
                tunnel: w575 -> [w587 _]
                tunnel: [w583 w631] -> w568
                frame False {
                  w584 = 1 ("Avg")
                  # "Not there yet."
                  n297 = Add(x=w595, y=w594) -> (x+y=w609:i32)
                  n298 = Quotient & Remainder(x=w609, y=2) -> (floor(x/y)=w583:i32)  [unwired: 1 out]
                  n299 = local write "DAC Value"(w583) -> ()
                  n300 = call <instrlib>:"Set DAC.vi"("error in (no error)"=w607, "value (0)"=w583, "chan (0)"=w588, "VISA resource name"=w587) -> ("error out"=w606:errorcluster, "VISA resource name out"=w603:refnum<visa-resource-name>)  [unwired: 6 in]
                  n301 = call <userlib>:"Wait (ms)__ogtk.vi"("error in (no error)"=w606, "milliseconds to wait"=u32 5) -> ("error out"=w604:errorcluster)  [unwired: 8 in, 1 out]
                  n302 = local read "Oversample"() -> (w602:i32)
                  n303 = for {
                    N: w584 -> [_]
                    tunnel: w603 -> [w614]
                    tunnel: [w612] -> w601 mode=indexing
                    tunnel: w588 -> [w610]
                    shift-right: [w611] -> w590
                    shift-left: w604 -> [w615]
                    w613 = u16 0 items=["High", "Med", "Low"] ("Gain")
                    n304 = call <instrlib>:"Get ADC.vi"("Gain"=w613, "Detector"=w610, "error in (no error)"=w615, "VISA resource name"=w614) -> ("error out"=w611:errorcluster, "output"=w612:i32)  [unwired: 5 in, 1 out]
                  }
                  n305 = Add Array Elements(numeric array=w601) -> (sum=w586:i32)
                  n306 = Divide(x=w586, y=w584) -> (x/y=w585:dbl)
                  n307 = Divide(x=w585, y=w602) -> (x/y=w589:dbl)
                  n308 = Subtract(x=w589, y="Target Counts") -> (x-y=w592:dbl)
                  n309 = local write "Counts"(w589) -> ()
                  n310 = Absolute Value(x=w592) -> (abs(x)=w599:dbl)
                  n311 = Less?(x=w599, y="Tolerance") -> (x < y?=w597:bool)
                  n312 = case shown="True" w597 {
                    tunnel: [FALSE TRUE] -> w596
                    tunnel: w583 -> [w619 w629]
                    tunnel: w595 -> [w620 w628]
                    tunnel: w594 -> [w618 _]
                    tunnel: [w616 w629] -> w593
                    tunnel: w592 -> [w622 _]
                    tunnel: [w617 w628] -> w591
                    frame False {
                      # "Not there, so examine difference\nbetween target and reading"
                      n313 = Greater Than 0?(x=w622) -> (x > 0?=w621:bool)
                      n314 = case shown="False" w621 {
                        tunnel: w620 -> [_ w627]
                        tunnel: w619 -> [w625 w626]
                        tunnel: w618 -> [w624 _]
                        tunnel: [w625 w627] -> w617
                        tunnel: [w624 w626] -> w616
                        frame False {
                          # "Reading is below target, so next DAC vaue will be below midpoint"
                        }
                        frame True {
                          # "If reading is above target, then next DAC value will be above mid"
                        }
                      }
                    }
                    frame True {
                      # "Within tolerance, so finish"
                    }
                  }
                }
                frame True {
                  # "DAC Values identical so finish"
                }
              }
              n315 = property on="Counts" class="WFChart (strict)"(error in=w566) -> (error out=w565:errorcluster, "Value"=w564:dbl)  [unwired: 1 in, 1 out]
              n316 = To Double Precision Float(number=w569) -> (double precision float=w572:dbl)
              n317 = To Double Precision Float(number=w568) -> (double precision float=w567:dbl)
              n318 = To Double Precision Float(number=w570) -> (double precision float=w571:dbl)
            }
            n319 = Build Array(w555, w554, w550, w553) -> (w552:dbl[][])
            n320 = property on="Searching..." class="Bool (strict)"(error in=w559, "Value"=FALSE ("Searching...")) -> ()  [unwired: 1 in, 2 out]
            n321 = Transpose 2D Array(2D array=w552) -> (transposed array=→"Searching":dbl[][])
          }
          event "Exit": Value Change {
            # "If stage is connected, go to reference position and then exit"
            n322 = event-data() -> ()  [unwired: 1 in, 6 out]
          }
          event Panel Close? {
            # "Discard \"Panel Close?\" event\n\nto leave program through\n graceful route"
            # "NOTE:\nMake sure not to use the red \"Abort Execution\" button in the\nLabVIEW menu to abort the application execution.\nDoing so will not close the device connection with the consequence that\na re-open after the next application start will fail."
            # "\"Panel Close\" (\"X\") was clicked by the user:\nWe discard the close command and set an \"exit\" flag. This gives us the change to proper disconnect the device and clean up the application before closing the window."
            # "Trap \"Panel Close\" instruction and exit program gracefully"
            n323 = event-data() -> ()  [unwired: 1 in, 4 out]
            n324 = local write "exit"(TRUE ("exit")) -> ()
            n325 = event-data("Discard?"=TRUE) -> ()  [unwired: 1 in, 1 out]
          }
        }
      }
    }
    frame #2 {
      # "Also power off and close detector SCPI EGSE"
      # "Cleanup and Shutdown"
      n326 = local read "Detector Resource"() -> (w643:refnum<visa-resource-name>)
      n327 = call <instrlib>:"Set Power.vi"("Power (0)"=FALSE, "VISA resource name"=w643) -> ("error out"=w640:errorcluster, "VISA resource name out"=w644:refnum<visa-resource-name>)  [unwired: 8 in]
      n328 = property on="Power" class="Bool (strict)"(error in=w640, "Value"=FALSE ("Power")) -> (error out=w641:errorcluster)  [unwired: 1 in, 1 out]
      n329 = call <instrlib>:"Close.vi"("error in (no error)"=w641, "VISA resource name"=w644) -> ("error out"=w638:errorcluster)  [unwired: 9 in]
      n330 = local read "PicoAmmeter Resource"() -> (w637:refnum<visa-resource-name>)
      n331 = call <instrlib>:"Close.vi"("error in (no error)"=w638, "VISA resource name"=w637) -> ()  [unwired: 9 in, 1 out]
    }
  }
  "error out" <- w1
